vi "Check if Date Matches File Name.vi"(8 "error in":errorcluster, 10 "DateTime Out":timestamp, 11 "Image Path":path) -> (0 "error out":errorcluster, 2 "resulting string":string, 3 "Date matches file name":bool)   [LabVIEW 2018, in "Main.lvlib"]
uses:
  Main.lvlib
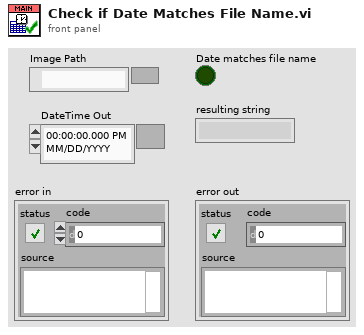
[diagram p1: front panel]
types:
  T1 = typedef "LVDateTimeRec.ctl" = cluster{"fractional second":dbl, "second":i32, "minute":i32, "hour":i32, "day of month":i32, "month":i32, "year":i32, "day of week":i32, "day of year":i32, "DST":i32}
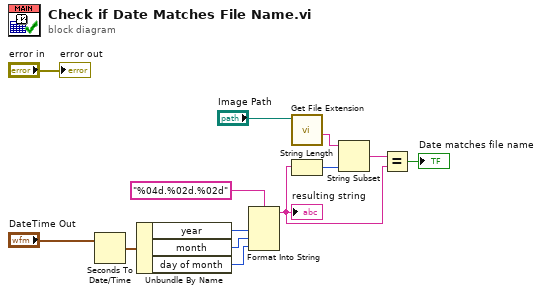
[diagram p0: block diagram]
diagram:
  n1 = Seconds To Date/Time(time stamp (now)="DateTime Out") -> (date time rec=w2:T1)  [unwired: 1 in]
  n2 = Unbundle By Name(w2) -> ("year"=w8:i32, "month"=w9:i32, "day of month"=w10:i32)
  n3 = Format Into String(format string="%04d.%02d.%02d", w8, w9, w10) -> (resulting string=w6:string)  [unwired: 2 in, 1 out]
  "resulting string" <- w6
  n4 = call <vilib>:"Get File Extension.vi"("file"="Image Path") -> ("filename without extension"=w11:string)  [unwired: 6 in, 4 out]
  n5 = String Length(string=w6) -> (length=w4:i32)
  n6 = String Subset(string=w11, length (rest)=w4) -> (substring=w5:string)  [unwired: 1 in]
  n7 = Equal?(x=w5, y=w6) -> (x = y?=→"Date matches file name":bool)
  "error out" <- "error in"
